vi "FissionReactorMultiblock.vi"(7 "Reactor Build Properties":T2, 8 "Biome Temperature":dbl=0.8, 9 "Fuel Input (mB/t)":i64, 10 "Burn Rate (mB/t)":dbl, 11 "Port States In":T1) -> (3 "Port States Out":T1, 4 "Temperature (K)":dbl, 6 "Heating Rate (mB/t)":i64)   [LabVIEW 2026]
uses:
  Fission Reactor Build Properties.ctl
  Port Defs/Reactor Port States.ctl
panel:
  out "x-y":dbl
  out "fuel":i64
  out "x+y":dbl format="%.2f"
  in  "x":dbl=1.0
  out "Steam Tank Pressure (bar)":dbl(knob) scale=0.0..65.0 scale format="%#_6p"
  out "Water Pressure (bar)":dbl(knob) scale=0.0..100.0
  out "Meltdown":bool
  out "Damage":dbl
  out "toBurn":dbl
  out "Reactor Stats":dbl(graph)
  out "Cooled Coolant Tank (mB)":i64(slide) scale=-1.0..21600000.0
  out "Heated Coolant Tank (mB)":i64(slide) scale=-1.0..216000000.0
  out "Emitted Waste (mB/t)":i64
  out "Waste Tank (mB)":i64(slide) scale=-1.0..192000.0
  out "Fissile Fuel Tank (mB)":i64(slide) scale=-1.0..192000.0
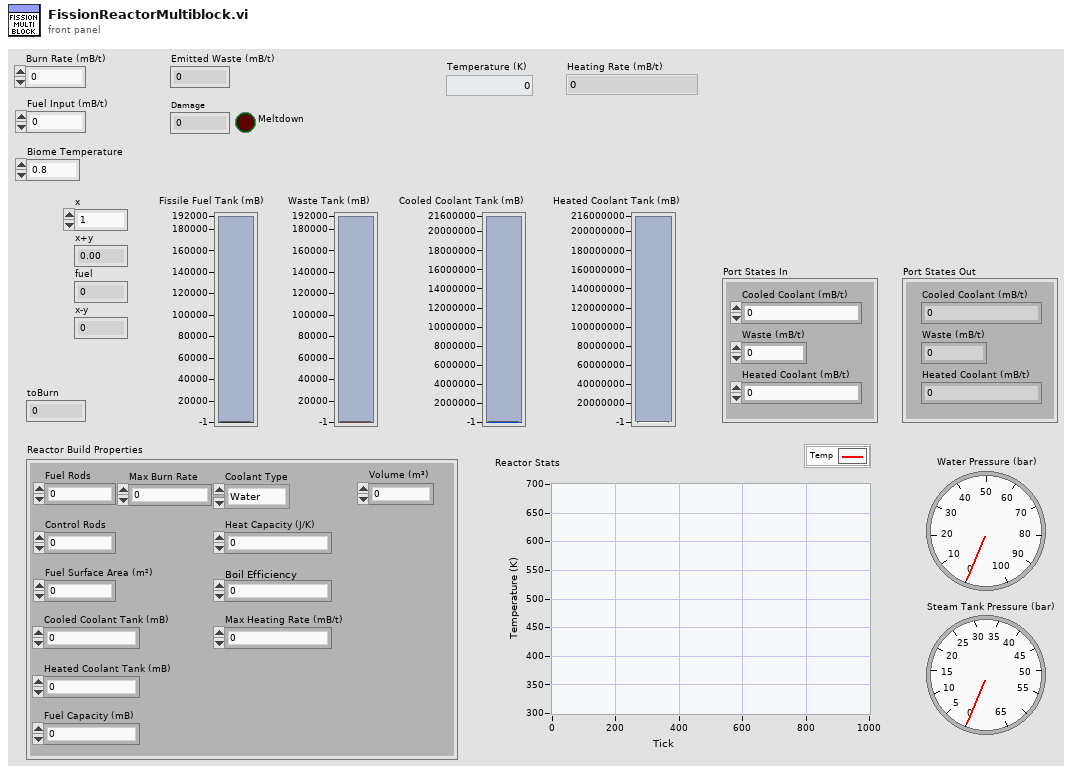
[diagram p1: front panel]
types:
  T1 = typedef "Reactor Port States.ctl" = cluster{"Cooled Coolant (mB/t)":i64, "Waste (mB/t)":i64, "Heated Coolant (mB/t)":i64}
  T2 = typedef "Fission Reactor Build Properties.ctl" = cluster{"Fuel Rods":i32, "Control Rods":i32, "Volume (m³)":i32, "Fuel Surface Area (m²)":i32, "Cooled Coolant Tank (mB)":i32, "Fuel Capacity (mB)":i64, "Heat Capacity (J/K)":dbl, "Max Burn Rate":i64, "Max Heating Rate (mB/t)":i64, "Boil Efficiency":dbl, "Coolant Type":enum16{"Water", "Sodium"}, "Heated Coolant Tank (mB)":i64}
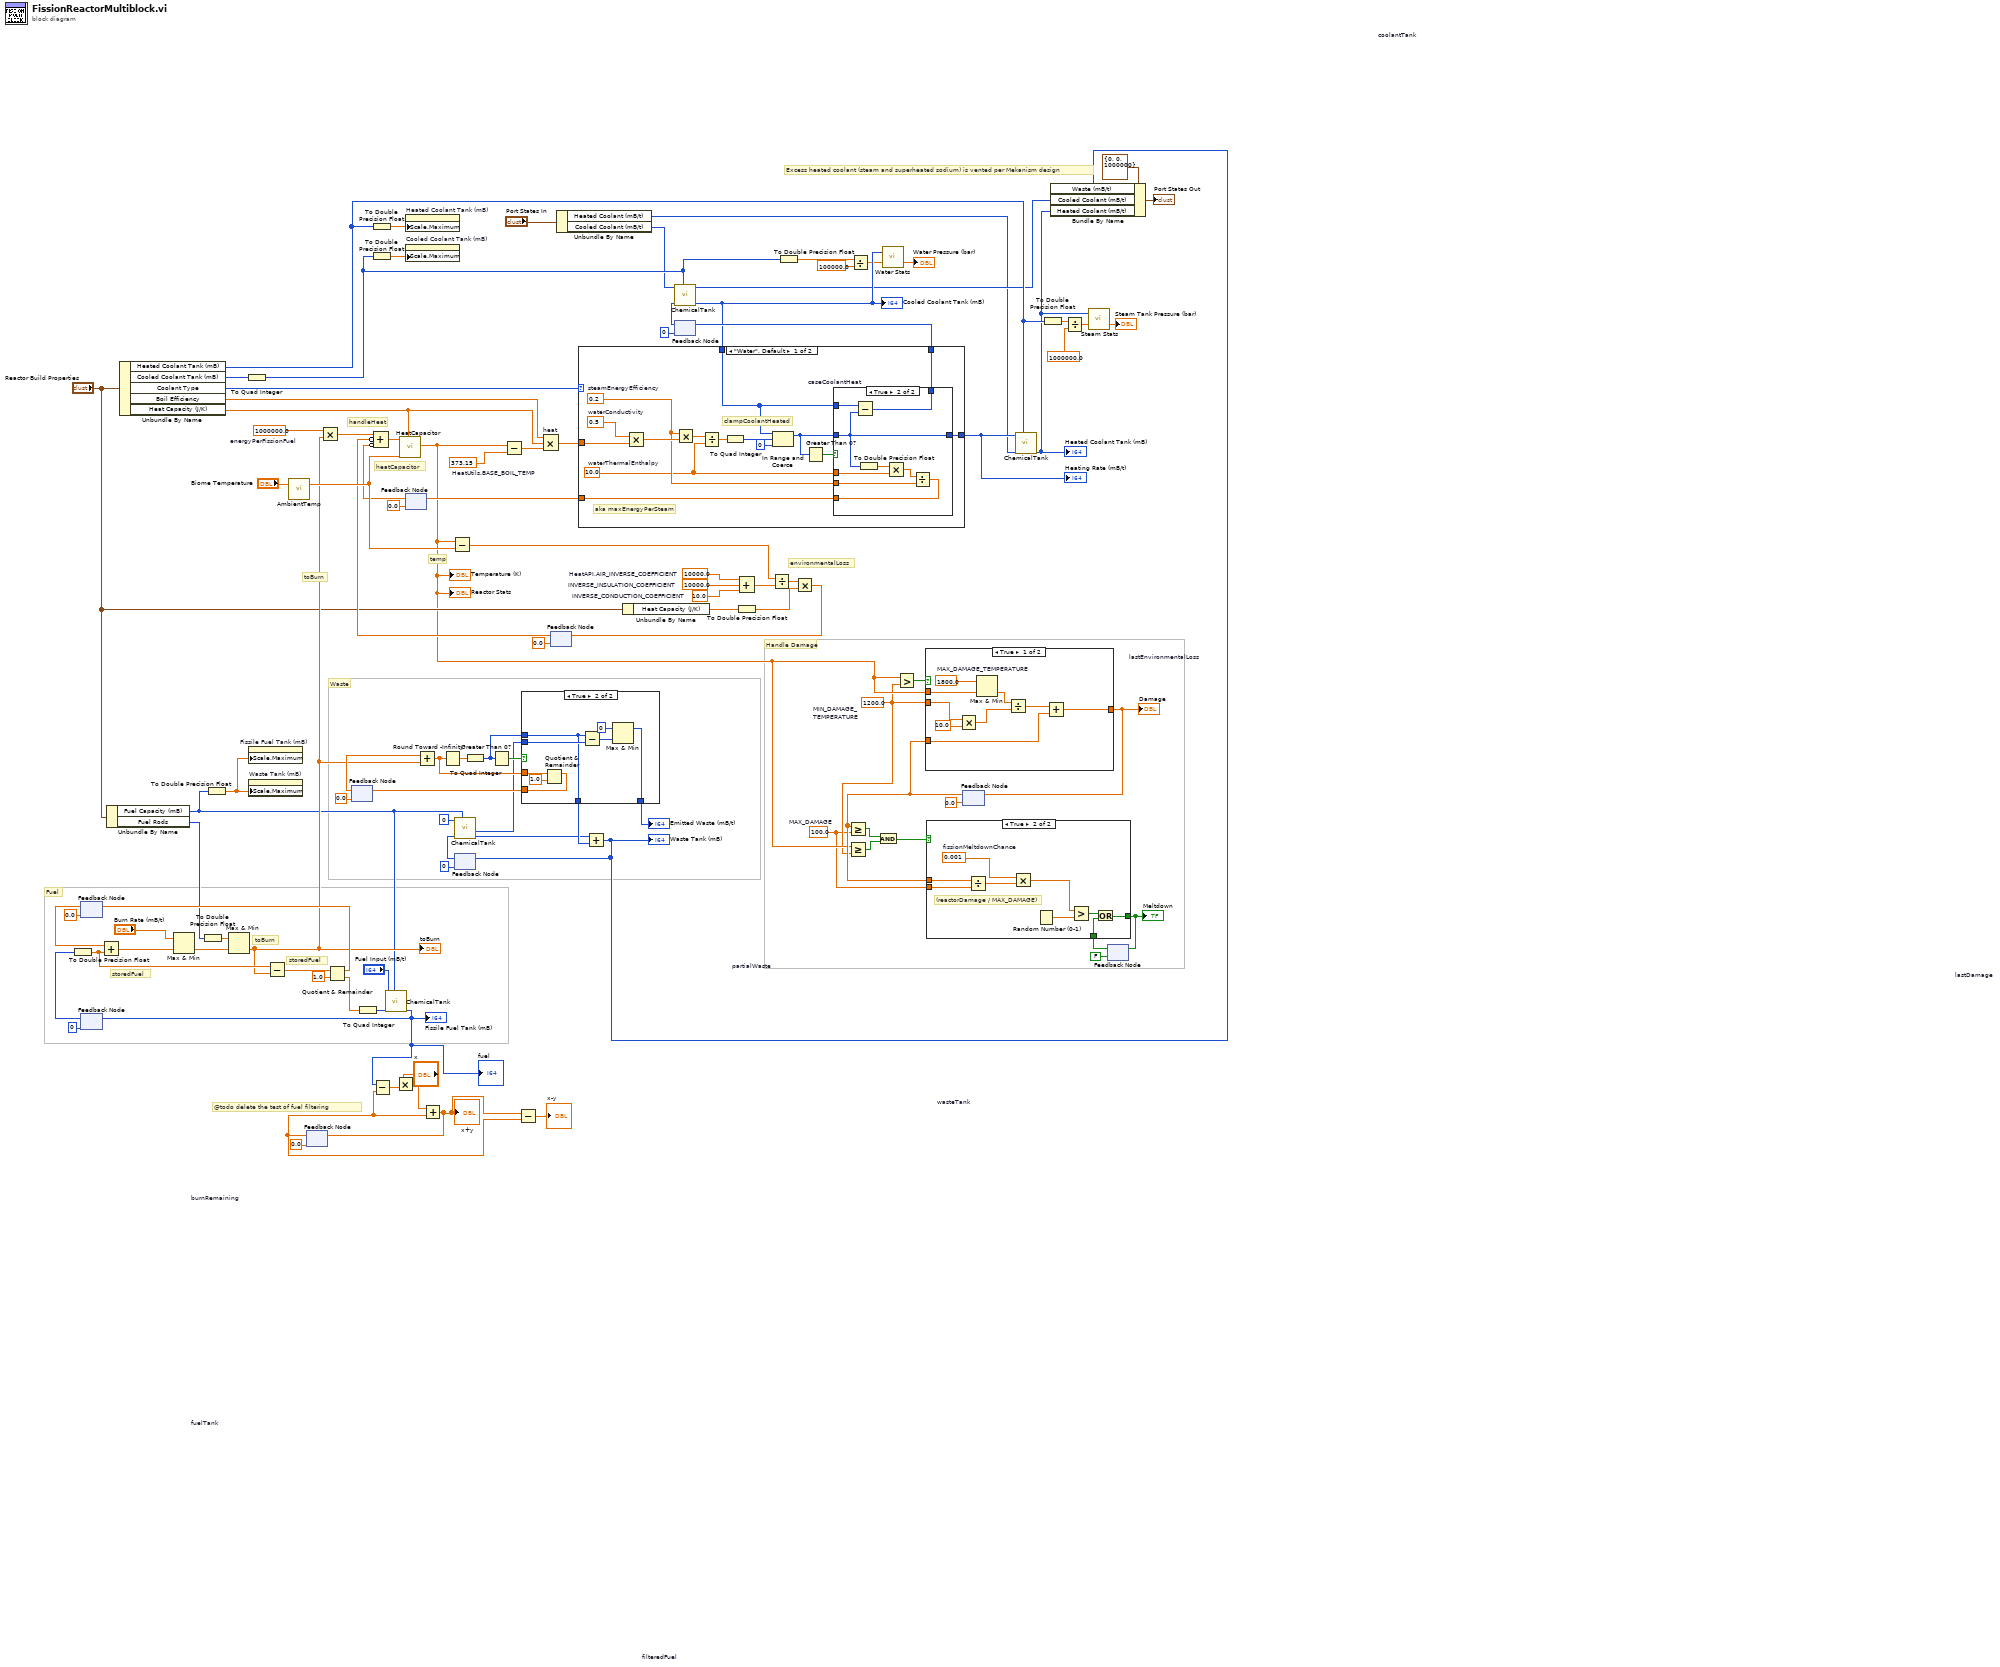
[diagram p0: block diagram]
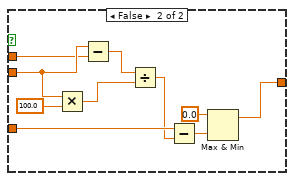
[diagram p3: hidden frame]
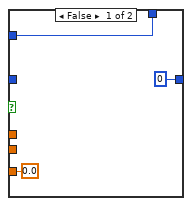
[diagram p4: hidden frame]
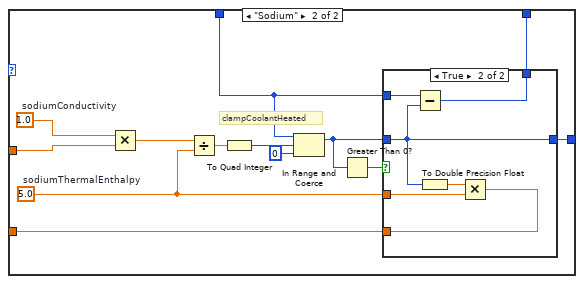
[diagram p5: hidden frame]
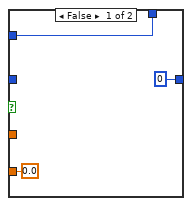
[diagram p6: hidden frame]
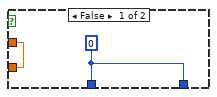
[diagram p7: hidden frame]
diagram:
  w32 = 100.0  # MAX_DAMAGE
  w33 = 1200.0  # MIN_DAMAGE_TEMPERATURE
  w63 = 10.0  # INVERSE_CONDUCTION_COEFFICIENT
  w64 = 10000.0  # INVERSE_INSULATION_COEFFICIENT
  w65 = 10000.0  # HeatAPI.AIR_INVERSE_COEFFICIENT
  w75 = 373.15  # HeatUtils.BASE_BOIL_TEMP
  w87 = 1000000.0  # energyPerFissionFuel
  # "@todo delete the test of fuel filtering"
  # "Handle Damage"
  # "Excess heated coolant (steam and superheated sodium) is vented per Mekanism design"
  # "handleHeat"
  # "toBurn"
  # "temp"
  # "environmentalLoss"
  # "Waste"
  # "heatCapacitor"
  # "Fuel"
  # "storedFuel"
  # "storedFuel"
  # "toBurn"
  n1 = feedback #1 "burnRemaining"(0.0) -> (w100:dbl)
  n2 = feedback #2 "fuelTank"(i64 0) -> (w101:i64)
  n3 = To Double Precision Float(number=w101) -> (double precision float=w95:dbl)
  n4 = Add(x=w100, y=w95) -> (x+y=w99:dbl)
  n5 = Unbundle By Name("Reactor Build Properties") -> ("Fuel Capacity (mB)"=w42:i64, "Fuel Rods"=w83:i32)
  n6 = Unbundle By Name("Reactor Build Properties") -> ("Heated Coolant Tank (mB)"=w20:i64, "Cooled Coolant Tank (mB)"=w49:i32, "Coolant Type"=w55:enum16{"Water", "Sodium"}, "Boil Efficiency"=w53:dbl, "Heat Capacity (J/K)"=w45:dbl)
  n7 = Max & Min(x="Burn Rate (mB/t)", y=w99) -> (min(x,y)=w97:dbl)  [unwired: 1 out]
  n8 = To Double Precision Float(number=w83) -> (double precision float=w96:dbl)
  n9 = To Double Precision Float(number=w42) -> (double precision float=w48:dbl)
  n10 = Max & Min(x=w96, y=w97) -> (min(x,y)=w88:dbl)  [unwired: 1 out]
  "toBurn" <- w88
  n11 = To Quad Integer(1:w49) -> (0:w25:i64)
  n12 = property on="Fissile Fuel Tank (mB)" class="Slide (strict)"("Scale.Maximum"=w48) -> ()  [unwired: 2 in, 2 out]
  n13 = property on="Waste Tank (mB)" class="Slide (strict)"("Scale.Maximum"=w48) -> ()  [unwired: 2 in, 2 out]
  n14 = Subtract(x=w95, y=w88) -> (x-y=w93:dbl)
  n15 = call "AmbientTemp.vi"("Biome Temperature"="Biome Temperature") -> ("Biome Ambient Temp (K)"=w105:dbl)  [unwired: 18 in]
  n16 = feedback #3 "filteredFuel"(0.0) -> (w2:dbl)
  n17 = Multiply(x=w87, y=w88) -> (x*y=w72:dbl)
  n18 = Quotient & Remainder(x=w93, y=1.0) -> (x-y*floor(x/y)=w92:dbl, floor(x/y)=w8:dbl)
  n19 = feedback-in #1(w92) -> ()
  n20 = feedback #4 "partialWaste"(0.0) -> (w91:dbl)
  n21 = To Quad Integer(1:w8) -> (0:w43:i64)
  n22 = To Double Precision Float(number=w20) -> (double precision float=w47:dbl)
  n23 = To Double Precision Float(number=w25) -> (double precision float=w46:dbl)
  n24 = call "ChemicalTank.vi"("Capacity (mB)"=w42, "Last Fill (mB)"=w43, "Transfer (mB)"="Fuel Input (mB/t)") -> ("Fill (mB)"=w3:i64)  [unwired: 2 in, 3 out]
  "Fissile Fuel Tank (mB)" <- w3
  "fuel" <- w3
  n25 = feedback-in #2(w3) -> ()
  n26 = Subtract(x=w3, y=w2) -> (x-y=w7:dbl)
  n27 = Multiply(x="x", y=w7) -> (x*y=w5:dbl)
  n28 = feedback #5 "caseCoolantHeat"(0.0) -> (w60:dbl)
  n29 = property on="Heated Coolant Tank (mB)" class="Slide (strict)"("Scale.Maximum"=w47) -> ()  [unwired: 2 in, 2 out]
  n30 = property on="Cooled Coolant Tank (mB)" class="Slide (strict)"("Scale.Maximum"=w46) -> ()  [unwired: 2 in, 2 out]
  n31 = Add(x=w91, y=w88) -> (x+y=w85:dbl)
  n32 = Add(x=w5, y=w2) -> (x+y=w4:dbl)
  "x+y" <- w4
  n33 = feedback-in #3(w4) -> ()
  n34 = Round Toward -Infinity(1:w85) -> (0:w89:dbl)
  n35 = feedback #6 "wasteTank"(i64 0 ("Fill (mB)")) -> (w82:i64)
  n36 = call "ChemicalTank.vi"("Capacity (mB)"=w42, "Last Fill (mB)"=w82, "Transfer (mB)"=i64 0 ("Input (mB)")) -> ("Fill (mB)"=w77:i64, "Needed (mB)"=w80:i64)  [unwired: 2 in, 2 out]
  n37 = To Quad Integer(1:w89) -> (0:w79:i64)
  n38 = Greater Than 0?(x=w79) -> (x > 0?=w86:bool)
  n39 = Subtract(x=w4, y=w2) -> (x-y=→"x-y":dbl)
  n40 = case shown="True" w86 {
    tunnel: w85 -> [w108 w115]
    tunnel: [w108 w114] -> w84
    tunnel: w80 -> [_ w113]
    tunnel: w79 -> [_ w110]
    tunnel: [w107 w110] -> w78
    tunnel: [w107 w109] -> w41
    frame False {
      w107 = i64 0
    }
    frame True {
      n41 = Quotient & Remainder(x=w115, y=1.0) -> (x-y*floor(x/y)=w114:dbl)  [unwired: 1 out]
      n42 = Subtract(x=w110, y=w113) -> (x-y=w112:i64)
      n43 = Max & Min(x=i64 0, y=w112) -> (max(x,y)=w109:i64)  [unwired: 1 out]
    }
  }
  "Emitted Waste (mB/t)" <- w41
  n44 = feedback-in #4(w84) -> ()
  n45 = feedback #7 "lastEnvironmentalLoss"(0.0) -> (w58:dbl)
  n46 = Compound Arithmetic op=ADD(w72, invert w58, invert w60) -> (w71:dbl)
  n47 = call "HeatCapacitor.vi"("Capacity (J/K)"=w45, "Ambient Temperature (K)"=w105, "Transfer (J)"=w71) -> ("Temperature (K)"=w37:dbl)  [unwired: 7 in, 1 out]
  "Temperature (K)" <- w37
  "Reactor Stats" <- w37
  n48 = Subtract(x=w37, y=w105) -> (x-y=w62:dbl)
  n49 = Subtract(x=w37, y=w75) -> (x-y=w54:dbl)
  n50 = Compound Arithmetic op=MULTIPLY "heat"(w53, w45, w54) -> (w74:dbl)
  n51 = Unbundle By Name("Port States In") -> ("Heated Coolant (mB/t)"=w12:i64, "Cooled Coolant (mB/t)"=w13:i64)
  n52 = Add(x=w77, y=w78) -> (x+y=w106:i64)
  "Waste Tank (mB)" <- w106
  n53 = feedback-in #6(w106) -> ()
  n54 = Unbundle By Name("Reactor Build Properties") -> ("Heat Capacity (J/K)"=w52:dbl)
  n55 = feedback #8 "coolantTank"(i64 0 ("Fill (mB)")) -> (w67:i64)
  n56 = call "ChemicalTank.vi"("Capacity (mB)"=w25, "Last Fill (mB)"=w67, "Transfer (mB)"=w13) -> ("Fill (mB)"=w28:i64, "Overflow (mB)"=w14:i64)  [unwired: 2 in, 2 out]
  "Cooled Coolant Tank (mB)" <- w28
  n57 = case shown="\"Water\", Default" w55 {
    tunnel: w74 -> [w131 w155]
    tunnel: w28 -> [w118 w144]
    tunnel: [w119 w146] -> w73
    tunnel: [w123 w150] -> w70
    tunnel: [w117 w143] -> w68
    frame "Water", Default {
      w122 = 10.0  # waterThermalEnthalpy
      w124 = 0.2  # steamEnergyEfficiency
      w130 = 0.5  # waterConductivity
      # "aka maxEnergyPerSteam"
      # "clampCoolantHeated"
      n58 = Multiply(x=w130, y=w131) -> (x*y=w129:dbl)
      n59 = Multiply(x=w124, y=w129) -> (x*y=w128:dbl)
      n60 = Divide(x=w128, y=w122) -> (x/y=w127:dbl)
      n61 = To Quad Integer(1:w127) -> (0:w126:i64)
      n62 = In Range and Coerce(upper limit=w118, x=w126, lower limit=i64 0) -> (coerced(x)=w120:i64)  [unwired: 1 out]
      n63 = Greater Than 0?(x=w120) -> (x > 0?=w121:bool)
      n64 = case shown="True" w121 {
        tunnel: w120 -> [_ w136]
        tunnel: w122 -> [_ w141]
        tunnel: w124 -> [_ w139]
        tunnel: [0.0 w138] -> w123
        tunnel: [i64 0 ("Fill (mB)") w136] -> w119
        tunnel: w118 -> [w132 w137]
        tunnel: [w132 w135] -> w117
        frame False {
        }
        frame True {
          n65 = Subtract(x=w137, y=w136) -> (x-y=w135:i64)
          n66 = To Double Precision Float(number=w136) -> (double precision float=w142:dbl)
          n67 = Multiply(x=w142, y=w141) -> (x*y=w140:dbl)
          n68 = Divide(x=w140, y=w139) -> (x/y=w138:dbl)
        }
      }
    }
    frame "Sodium" {
      w149 = 5.0  # sodiumThermalEnthalpy
      w154 = 1.0  # sodiumConductivity
      # "clampCoolantHeated"
      n69 = Multiply(x=w154, y=w155) -> (x*y=w145:dbl)
      n70 = Divide(x=w145, y=w149) -> (x/y=w153:dbl)
      n71 = To Quad Integer(1:w153) -> (0:w152:i64)
      n72 = In Range and Coerce(upper limit=w144, x=w152, lower limit=i64 0) -> (coerced(x)=w147:i64)  [unwired: 1 out]
      n73 = Greater Than 0?(x=w147) -> (x > 0?=w148:bool)
      n74 = case shown="True" w148 {
        tunnel: w147 -> [_ w161]
        tunnel: w149 -> [_ w163]
        tunnel: [0.0 w162] -> w150
        tunnel: [i64 0 ("Fill (mB)") w161] -> w146
        tunnel: w144 -> [w156 w160]
        tunnel: [w156 w159] -> w143
        frame False {
        }
        frame True {
          n75 = Subtract(x=w160, y=w161) -> (x-y=w159:i64)
          n76 = To Double Precision Float(number=w161) -> (double precision float=w164:dbl)
          n77 = Multiply(x=w164, y=w163) -> (x*y=w162:dbl)
        }
      }
    }
  }
  "Heating Rate (mB/t)" <- w73
  n78 = feedback-in #5(w70) -> ()
  n79 = feedback-in #8(w68) -> ()
  n80 = To Double Precision Float(number=w52) -> (double precision float=w51:dbl)
  n81 = Compound Arithmetic op=unknown(w65, w64, w63) -> (w61:dbl)
  n82 = Divide(x=w62, y=w61) -> (x/y=w57:dbl)
  n83 = To Double Precision Float(number=w25) -> (double precision float=w18:dbl)
  n84 = Multiply(x=w57, y=w51) -> (x*y=w59:dbl)
  n85 = feedback-in #7(w59) -> ()
  n86 = Greater Or Equal?(x=w37, y=w33) -> (x >= y?=w35:bool)
  n87 = Divide(x=w18, y=100000.0) -> (x/y=w24:dbl)
  n88 = call "Water Stats.vi"("Divisor"=w24, "Flow"=w28) -> ("Pressure (bar)"=→"Water Pressure (bar)":dbl)  [unwired: 1 out]
  n89 = Greater?(x=w37, y=w33) -> (0:w39:bool)
  n90 = feedback #9 "lastDamage"(0.0) -> (w104:dbl)
  n91 = Greater Or Equal?(x=w104, y=w32) -> (x >= y?=w36:bool)
  n92 = And(x=w36, y=w35) -> (x .and. y?=w34:bool)
  n93 = case shown="True" w39 {
    tunnel: w33 -> [w172 w181]
    tunnel: w37 -> [w166 w180]
    tunnel: w104 -> [w168 w178]
    tunnel: [w167 w175] -> w38
    frame True {
      w165 = 1800.0  # MAX_DAMAGE_TEMPERATURE
      n94 = Multiply(x=w172, y=10.0) -> (x*y=w170:dbl)
      n95 = Max & Min(x=w165, y=w166) -> (min(x,y)=w173:dbl)  [unwired: 1 out]
      n96 = Divide(x=w173, y=w170) -> (x/y=w169:dbl)
      n97 = Add(x=w169, y=w168) -> (x+y=w167:dbl)
    }
    frame False {
      n98 = Multiply(x=w181, y=100.0) -> (x*y=w182:dbl)
      n99 = Subtract(x=w181, y=w180) -> (x-y=w179:dbl)
      n100 = Divide(x=w179, y=w182) -> (x/y=w177:dbl)
      n101 = Subtract(x=w178, y=w177) -> (x-y=w176:dbl)
      n102 = Max & Min(x=0.0, y=w176) -> (max(x,y)=w175:dbl)  [unwired: 1 out]
    }
  }
  "Damage" <- w38
  n103 = feedback-in #9(w38) -> ()
  n104 = call "ChemicalTank.vi"("Capacity (mB)"=w20, "Last Fill (mB)"=w12, "Transfer (mB)"=w73) -> ("Fill (mB)"=w15:i64)  [unwired: 2 in, 3 out]
  "Heated Coolant Tank (mB)" <- w15
  n105 = To Double Precision Float(number=w20) -> (double precision float=w19:dbl)
  n106 = Bundle By Name(cluster=T1 {"Cooled Coolant (mB/t)"=0, "Waste (mB/t)"=0, "Heated Coolant (mB/t)"=1000000} ("Port States Out"), "Waste (mB/t)"=w106, "Cooled Coolant (mB/t)"=w14, "Heated Coolant (mB/t)"=w15) -> (→"Port States Out":T1)
  n107 = Divide(x=w19, y=1000000.0) -> (x/y=w22:dbl)
  n108 = call "Steam Stats.vi"("Divisor"=w22, "Flow"=w15) -> ("Pressure (bar)"=→"Steam Tank Pressure (bar)":dbl)  [unwired: 1 out]
  n109 = feedback #10(FALSE) -> (w31:bool)
  n110 = case shown="True" w34 {
    tunnel: w104 -> [_ w192]
    tunnel: w32 -> [_ w191]
    tunnel: [w184 w186] -> w30
    tunnel: w31 -> [w184 w185]
    frame False {
    }
    frame True {
      w189 = 0.001  # fissionMeltdownChance
      # "(reactorDamage / MAX_DAMAGE)"
      n111 = Divide(x=w192, y=w191) -> (x/y=w190:dbl)
      n112 = Multiply(x=w189, y=w190) -> (x*y=w188:dbl)
      n113 = Random Number (0-1)() -> (number: 0 to 1=w193:dbl)
      n114 = Greater?(x=w188, y=w193) -> (0:w187:bool)
      n115 = Or(x=w187, y=w185) -> (x .or. y?=w186:bool)
    }
  }
  "Meltdown" <- w30
  n116 = feedback-in #10(w30) -> ()
